vi "Write Variant Cluster to Config File.vi"(5 "Index":i32, 7 "From Array?":bool, 8 "error in":errorcluster, 10 "Variant Configuration Object":variant, 11 "Config Refnum in":T1) -> (0 "error out":errorcluster, 3 "Config Refnum out":T1)   [LabVIEW 2018, in "EMS Generic Actor.lvlib" / "EMS Generic.lvclass"]
doc: "This VI accepts either a Cluster or Array of Clusters that has been converted to a variant. The label of the cluster is used to define the section name and individual control names are used to define key names."
uses:
  EMS Generic.lvclass
  <vilib>/Utility/config.llb/Config Data RefNum.ctl
  <vilib>/Utility/config.llb/Write Key (String).vi
  <vilib>/Utility/config.llb/Write Key (Double).vi
  <vilib>/Utility/config.llb/Write Key (U32).vi
  <vilib>/Utility/config.llb/Write Key (I32).vi
  <vilib>/Utility/config.llb/Write Key (Path).vi
  <vilib>/Utility/Data Type/NI_Data Type.lvlib
  <vilib>/Utility/config.llb/NI_LVConfig.lvlib
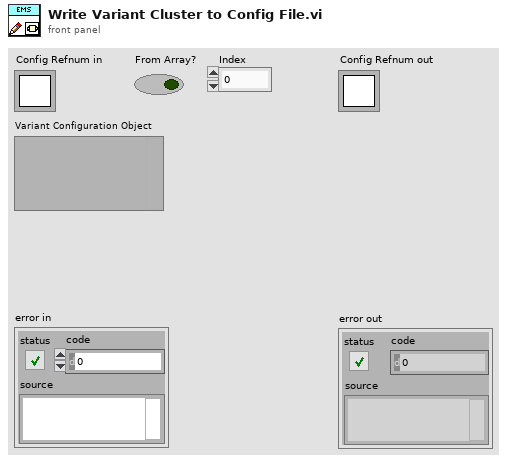
[diagram p1: front panel]
types:
  T1 = typedef "NI_LVConfig.lvlib/Config Data RefNum.ctl" = refnum<k1>
  T2 = typedef "NI_Data Type.lvlib/Data Type.ctl" = enum8{"Invalid Type", "Void", "I8", "I16", "I32", "I64", "U8", "U16", "U32", "U64", "Single Float", "Double Float", "Extended Float", "Single Complex", "Double Complex", "Extended Complex", "Enum U8", "Enum U16", "Enum U32", "Enum U64", "Single Float With Unit", "Double Float With Unit", "Extended Float With Unit", "Single Complex with Unit", "Double Complex with Unit", "Extended Complex with Unit", "Boolean", "String", "Path", "Picture", "Tag", "Array", "Cluster", "Variant", "LV Variant", "Waveform", "Timestamp", "Digital Waveform", "Digital Data", "ExpressData", "Refnum", "External Data", "VI", "Poly VI", "LabVIEW Class Instance", "Fixed Point"}
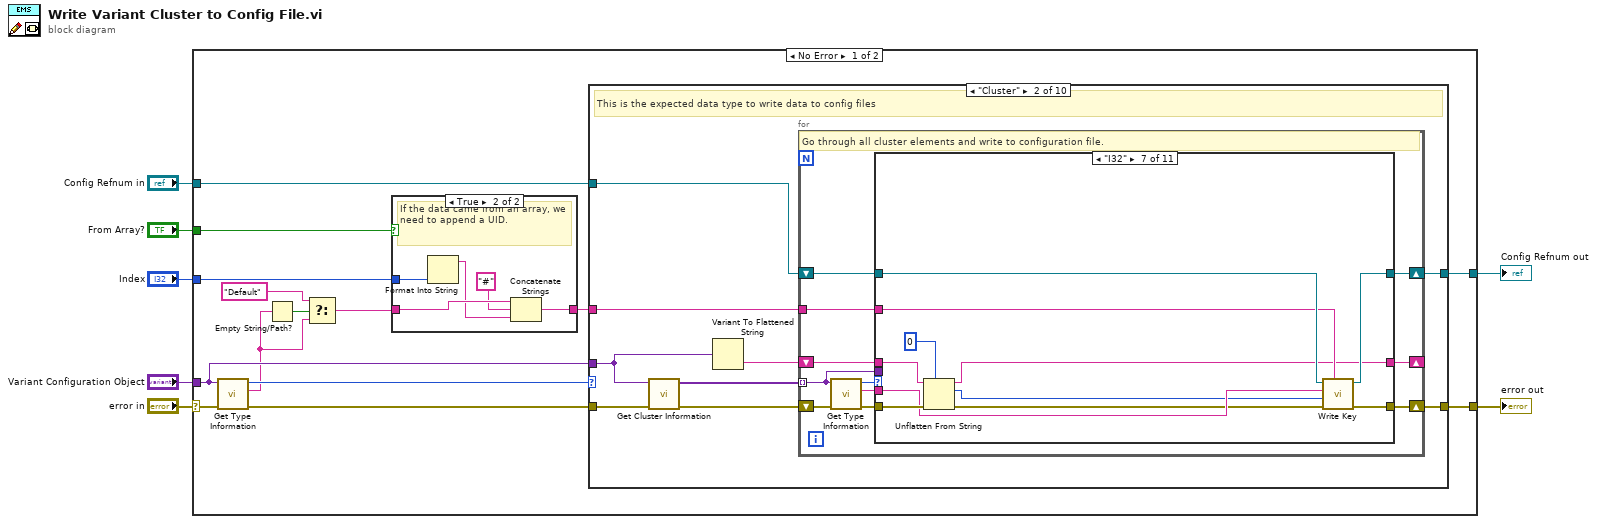
[diagram p0: block diagram]
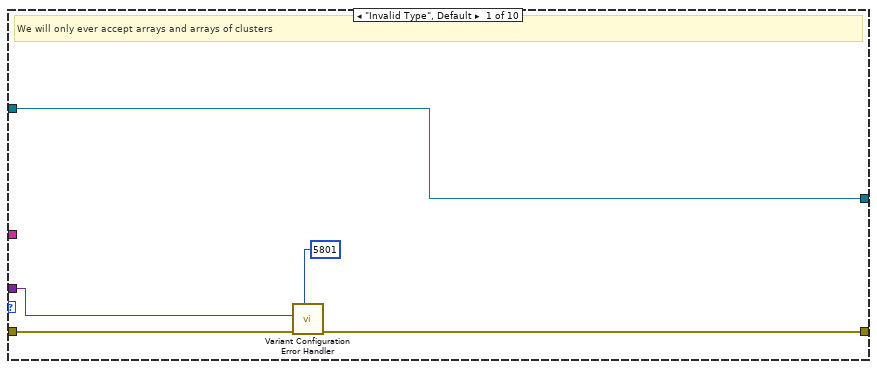
[diagram p2: hidden frame]
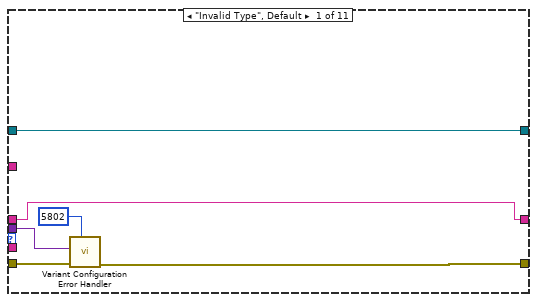
[diagram p3: hidden frame]
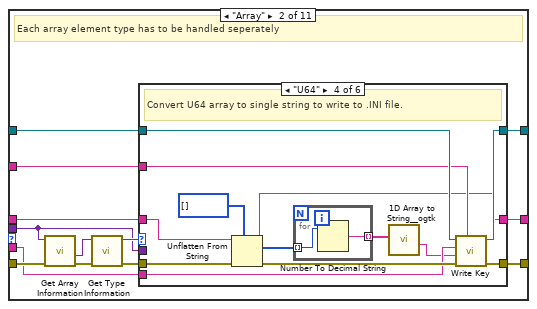
[diagram p4: hidden frame]
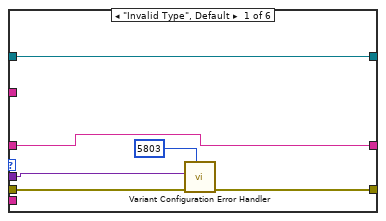
[diagram p5: hidden frame]
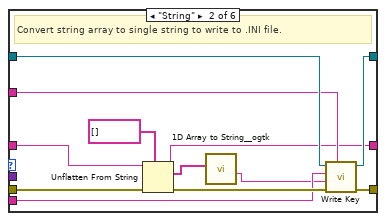
[diagram p6: hidden frame]
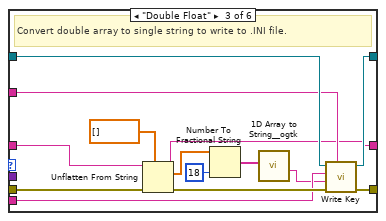
[diagram p7: hidden frame]
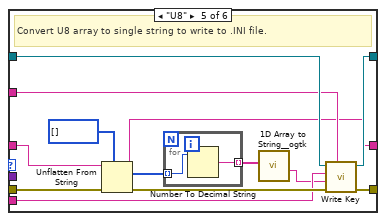
[diagram p8: hidden frame]
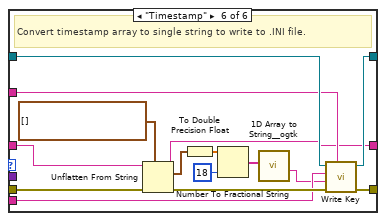
[diagram p9: hidden frame]
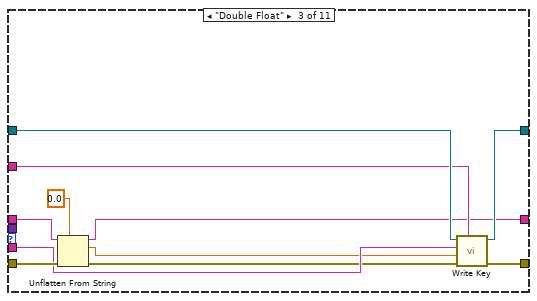
[diagram p10: hidden frame]
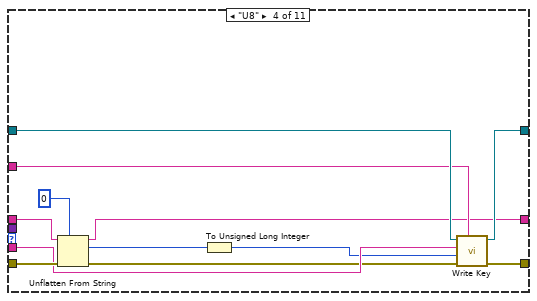
[diagram p11: hidden frame]
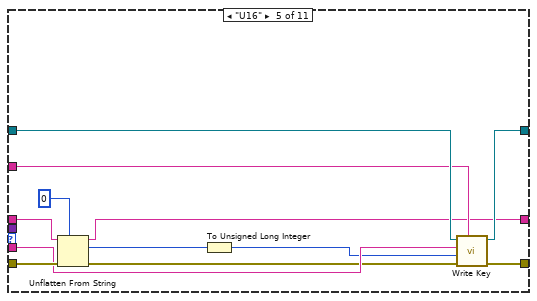
[diagram p12: hidden frame]
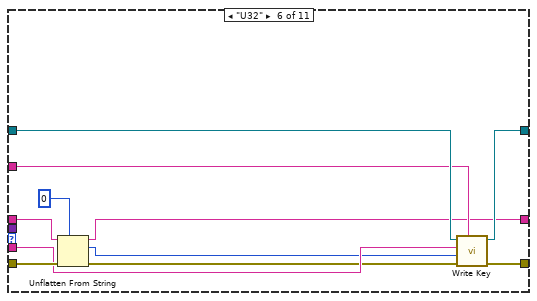
[diagram p13: hidden frame]
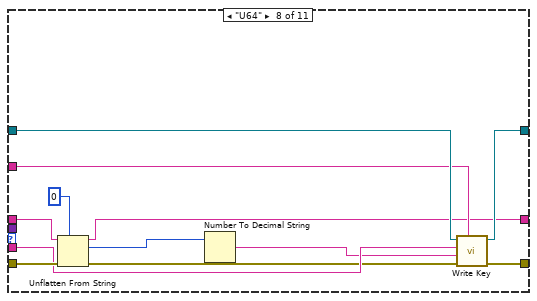
[diagram p14: hidden frame]
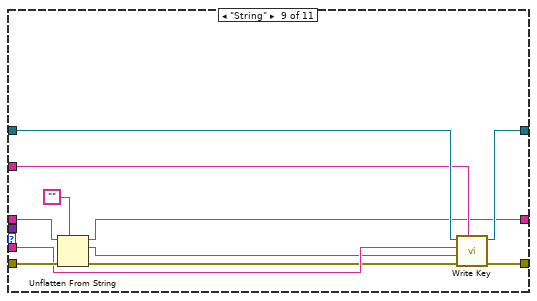
[diagram p15: hidden frame]
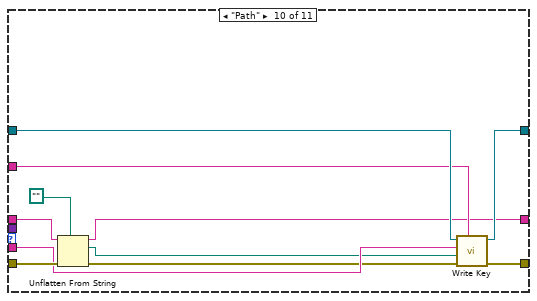
[diagram p16: hidden frame]
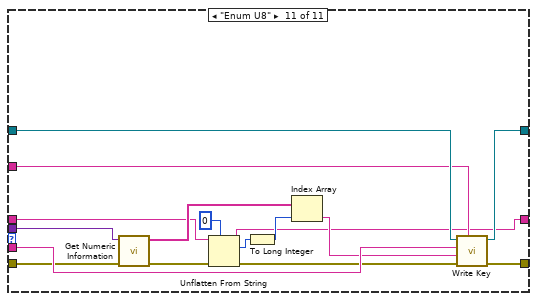
[diagram p17: hidden frame]
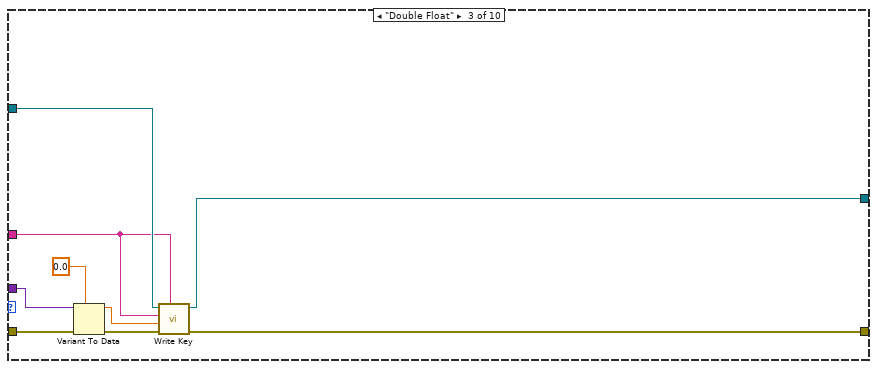
[diagram p18: hidden frame]
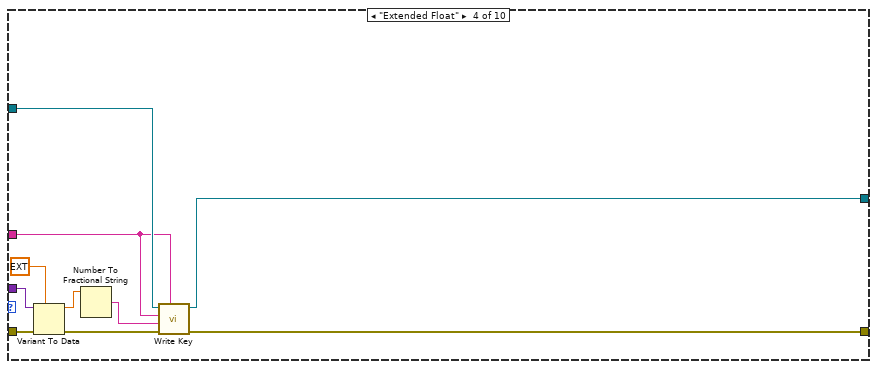
[diagram p19: hidden frame]
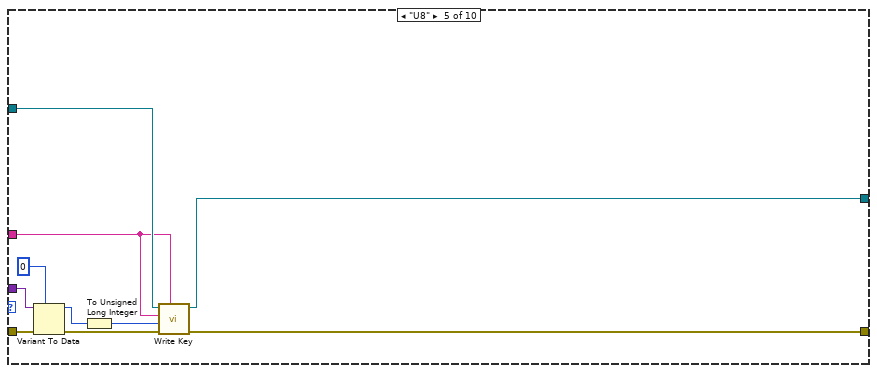
[diagram p20: hidden frame]
diagram:
  n1 = case shown="No Error" "error in" {
    selector: "error in" -> [w21 w340]
    tunnel: "Variant Configuration Object" -> [w19 _]
    tunnel: "Config Refnum in" -> [w17 w341]
    tunnel: "Index" -> [w13 _]
    tunnel: "From Array?" -> [w12 _]
    tunnel: [w16 w341] -> w2
    tunnel: [w15 w340] -> w1
    frame No Error {
      n2 = call <vilib>:"Get Type Information.vi"("error in (no error)"=w21, "Variant"=w19) -> ("error out"=w18:errorcluster, "Name"=w10:string, "Type"=w20:T2)  [unwired: 5 in, 2 out]
      n3 = Empty String/Path?(string/path=w10) -> (empty?=w11:bool)
      n4 = Select(t="Default", s=w11, f=w10) -> (s? t:f=w9:string)
      n5 = case shown="True" w12 {
        tunnel: w9 -> [w334 w338]
        tunnel: [w334 w335] -> w14
        tunnel: w13 -> [_ w339]
        frame False {
          # "Pass the name through as the section name."
        }
        frame True {
          # "If the data came from an array, we need to append a UID."
          n6 = Format Into String(w339) -> (resulting string=w336:string)  [unwired: 3 in, 1 out]
          n7 = Concatenate Strings(w338, "#" ("string"), w336) -> (w335:string)
        }
      }
      n8 = case shown="\"Cluster\"" w20 {
        tunnel: w19 -> [w24 w29 w255 w265 w275 w285 w294 w304 w313 w325]
        tunnel: w18 -> [w26 w35 w253 w263 w273 w283 w292 w302 w311 w326]
        tunnel: [w25 w33 w256 w266 w276 w286 w295 w305 w314 w320] -> w15
        tunnel: w17 -> [w22 w31 w258 w268 w278 w288 w297 w307 w316 w319]
        tunnel: [w22 w30 w257 w267 w277 w287 w296 w306 w315 w317] -> w16
        tunnel: w14 -> [_ w27 w250 w259 w269 w279 w289 w298 w308 _]
        frame "Invalid Type", Default {
          # "We will only ever accept arrays and arrays of clusters"
          n9 = call "Variant Configuration Error Handler.vi"("Error Code"=5801 ("error code (0)"), "error in"=w26, "Variant"=w24) -> ("error out"=w25:errorcluster)  [unwired: 8 in]
        }
        frame "Cluster" {
          # "This is the expected data type to write data to config files"
          n10 = call <vilib>:"Get Cluster Information.vi"("error in (no error)"=w35, "Variant"=w29) -> ("error out"=w34:errorcluster, "Cluster Elements"=w32:variant[])  [unwired: 8 in]
          n11 = Variant To Flattened String(Variant=w29) -> (data string=w28:string)  [unwired: 1 out]
          n12 = for {
            shift-right: [w43] -> w33
            shift-left: w34 -> [w46]
            tunnel: w32 -> [w36] mode=indexing
            tunnel: w27 -> [w41]
            shift-right: [w39] -> w30
            shift-left: w31 -> [w42]
            shift-right: [w37] -> _
            shift-left: w28 -> [w38]
            # "Go through all cluster elements and write to configuration file."
            n13 = call <vilib>:"Get Type Information.vi"("error in (no error)"=w46, "Variant"=w36) -> ("error out"=w44:errorcluster, "Name"=w40:string, "Type"=w45:T2)  [unwired: 5 in, 2 out]
            n14 = case shown="\"I32\"" w45 {
              tunnel: w44 -> [w51 w65 w153 w165 w177 w188 w199 w211 w222 w233 w242]
              tunnel: [w50 w58 w147 w159 w171 w182 w193 w204 w217 w228 w244] -> w43
              tunnel: w42 -> [w49 w60 w151 w163 w175 w186 w197 w209 w221 w232 w248]
              tunnel: w41 -> [_ w59 w150 w162 w174 w185 w196 w208 w220 w231 w247]
              tunnel: w40 -> [_ w57 w149 w161 w173 w184 w195 w207 w219 w230 w246]
              tunnel: [w49 w56 w146 w157 w169 w181 w192 w203 w216 w227 w243] -> w39
              tunnel: w38 -> [w48 w55 w144 w154 w166 w178 w189 w202 w215 w226 w235]
              tunnel: [w48 w54 w143 w155 w167 w179 w190 w201 w214 w225 w234] -> w37
              tunnel: w36 -> [w47 w53 _ _ _ _ _ _ _ _ w237]
              frame "Invalid Type", Default {
                n15 = call "Variant Configuration Error Handler.vi"("Error Code"=5802 ("error code (0)"), "error in"=w51, "Variant"=w47) -> ("error out"=w50:errorcluster)  [unwired: 8 in]
              }
              frame "Array" {
                # "Each array element type has to be handled seperately"
                n16 = call <vilib>:"Get Array Information.vi"("error in (no error)"=w65, "Variant"=w53) -> ("error out"=w63:errorcluster, "Array Element Data Type"=w62:variant)  [unwired: 6 in, 2 out]
                n17 = call <vilib>:"Get Type Information.vi"("error in (no error)"=w63, "Variant"=w62) -> ("error out"=w61:errorcluster, "Type"=w64:T2)  [unwired: 5 in, 3 out]
                n18 = case shown="\"U64\"" w64 {
                  tunnel: w61 -> [w70 w83 w97 w110 w125 w142]
                  tunnel: w60 -> [w68 w79 w93 w106 w121 w138]
                  tunnel: w59 -> [_ w78 w92 w105 w120 w137]
                  tunnel: [w69 w80 w94 w107 w122 w139] -> w58
                  tunnel: w57 -> [_ w77 w91 w104 w119 w136]
                  tunnel: [w68 w75 w87 w102 w117 w131] -> w56
                  tunnel: w55 -> [w67 w73 w85 w101 w116 w130]
                  tunnel: [w67 w72 w84 w100 w115 w128] -> w54
                  tunnel: w53 -> [w66 _ _ _ _ _]
                  frame "Invalid Type", Default {
                    n19 = call "Variant Configuration Error Handler.vi"("Error Code"=5803 ("error code (0)"), "error in"=w70, "Variant"=w66) -> ("error out"=w69:errorcluster)  [unwired: 8 in]
                  }
                  frame "String" {
                    # "Convert string array to single string to write to .INI file."
                    n20 = Unflatten From String(type=string[] [], binary string=w73, error in (no error)=w83) -> (rest of the binary string=w72:string, value=w74:string[], error out=w81:errorcluster)  [unwired: 2 in]
                    n21 = call <userlib>:"1D Array to String__ogtk.vi"("Array of Strings"=w74) -> ("delimited string"=w76:string)  [unwired: 10 in]
                    n22 = call-poly <vilib>:"Write Key.vi"("section"=w78, "error in (no error)"=w81, "value"=w76, "key"=w77, "refnum"=w79) -> ("error out"=w80:errorcluster, "refnum out"=w75:T1)  [unwired: 4 in, 1 out]
                  }
                  frame "Double Float" {
                    # "Convert double array to single string to write to .INI file."
                    n23 = Unflatten From String(type=dbl[] [], binary string=w85, error in (no error)=w97) -> (rest of the binary string=w84:string, value=w86:dbl[], error out=w95:errorcluster)  [unwired: 2 in]
                    n24 = Number To Fractional String(number=w86, precision (6)=i16 18) -> (F-format string=w89:string[])  [unwired: 2 in]
                    n25 = call <userlib>:"1D Array to String__ogtk.vi"("Array of Strings"=w89) -> ("delimited string"=w88:string)  [unwired: 10 in]
                    n26 = call-poly <vilib>:"Write Key.vi"("section"=w92, "error in (no error)"=w95, "value"=w88, "key"=w91, "refnum"=w93) -> ("error out"=w94:errorcluster, "refnum out"=w87:T1)  [unwired: 4 in, 1 out]
                  }
                  frame "U64" {
                    # "Convert U64 array to single string to write to .INI file."
                    n27 = Unflatten From String(type=u64[] [], binary string=w101, error in (no error)=w110) -> (rest of the binary string=w100:string, value=w99:u64[], error out=w108:errorcluster)  [unwired: 2 in]
                    n28 = for {
                      tunnel: w99 -> [w112] mode=indexing
                      tunnel: [w111] -> w98 mode=indexing
                      n29 = Number To Decimal String(number=w112) -> (decimal integer string=w111:string)  [unwired: 1 in]
                    }
                    n30 = call <userlib>:"1D Array to String__ogtk.vi"("Array of Strings"=w98) -> ("delimited string"=w103:string)  [unwired: 10 in]
                    n31 = call-poly <vilib>:"Write Key.vi"("section"=w105, "error in (no error)"=w108, "value"=w103, "key"=w104, "refnum"=w106) -> ("error out"=w107:errorcluster, "refnum out"=w102:T1)  [unwired: 4 in, 1 out]
                  }
                  frame "U8" {
                    # "Convert U8 array to single string to write to .INI file."
                    n32 = Unflatten From String(type=u8[] [], binary string=w116, error in (no error)=w125) -> (rest of the binary string=w115:string, value=w114:u8[], error out=w123:errorcluster)  [unwired: 2 in]
                    n33 = for {
                      tunnel: w114 -> [w127] mode=indexing
                      tunnel: [w126] -> w113 mode=indexing
                      n34 = Number To Decimal String(number=w127) -> (decimal integer string=w126:string)  [unwired: 1 in]
                    }
                    n35 = call <userlib>:"1D Array to String__ogtk.vi"("Array of Strings"=w113) -> ("delimited string"=w118:string)  [unwired: 10 in]
                    n36 = call-poly <vilib>:"Write Key.vi"("section"=w120, "error in (no error)"=w123, "value"=w118, "key"=w119, "refnum"=w121) -> ("error out"=w122:errorcluster, "refnum out"=w117:T1)  [unwired: 4 in, 1 out]
                  }
                  frame "Timestamp" {
                    # "Convert timestamp array to single string to write to .INI file."
                    n37 = Unflatten From String(type=timestamp[] [], binary string=w130, error in (no error)=w142) -> (rest of the binary string=w128:string, value=w129:timestamp[], error out=w140:errorcluster)  [unwired: 2 in]
                    n38 = To Double Precision Float(number=w129) -> (double precision float=w132:dbl[])
                    n39 = Number To Fractional String(number=w132, precision (6)=i16 18) -> (F-format string=w134:string[])  [unwired: 2 in]
                    n40 = call <userlib>:"1D Array to String__ogtk.vi"("Array of Strings"=w134) -> ("delimited string"=w133:string)  [unwired: 10 in]
                    n41 = call-poly <vilib>:"Write Key.vi"("section"=w137, "error in (no error)"=w140, "value"=w133, "key"=w136, "refnum"=w138) -> ("error out"=w139:errorcluster, "refnum out"=w131:T1)  [unwired: 4 in, 1 out]
                  }
                }
              }
              frame "Double Float" {
                n42 = Unflatten From String(type=0.0, binary string=w144, error in (no error)=w153) -> (rest of the binary string=w143:string, value=w145:dbl, error out=w148:errorcluster)  [unwired: 2 in]
                n43 = call-poly <vilib>:"Write Key.vi"("section"=w150, "error in (no error)"=w148, "value"=w145, "key"=w149, "refnum"=w151) -> ("error out"=w147:errorcluster, "refnum out"=w146:T1)  [unwired: 4 in, 1 out]
              }
              frame "U8" {
                n44 = Unflatten From String(type=u8 0, binary string=w154, error in (no error)=w165) -> (rest of the binary string=w155:string, value=w156:u8, error out=w160:errorcluster)  [unwired: 2 in]
                n45 = To Unsigned Long Integer(number=w156) -> (unsigned 32bit integer=w158:u32)
                n46 = call-poly <vilib>:"Write Key.vi"("section"=w162, "error in (no error)"=w160, "value"=w158, "key"=w161, "refnum"=w163) -> ("error out"=w159:errorcluster, "refnum out"=w157:T1)  [unwired: 4 in, 1 out]
              }
              frame "U16" {
                n47 = Unflatten From String(type=u16 0, binary string=w166, error in (no error)=w177) -> (rest of the binary string=w167:string, value=w168:u16, error out=w172:errorcluster)  [unwired: 2 in]
                n48 = To Unsigned Long Integer(number=w168) -> (unsigned 32bit integer=w170:u32)
                n49 = call-poly <vilib>:"Write Key.vi"("section"=w174, "error in (no error)"=w172, "value"=w170, "key"=w173, "refnum"=w175) -> ("error out"=w171:errorcluster, "refnum out"=w169:T1)  [unwired: 4 in, 1 out]
              }
              frame "U32" {
                n50 = Unflatten From String(type=u32 0, binary string=w178, error in (no error)=w188) -> (rest of the binary string=w179:string, value=w180:u32, error out=w183:errorcluster)  [unwired: 2 in]
                n51 = call-poly <vilib>:"Write Key.vi"("section"=w185, "error in (no error)"=w183, "value"=w180, "key"=w184, "refnum"=w186) -> ("error out"=w182:errorcluster, "refnum out"=w181:T1)  [unwired: 4 in, 1 out]
              }
              frame "I32" {
                n52 = Unflatten From String(type=0, binary string=w189, error in (no error)=w199) -> (rest of the binary string=w190:string, value=w191:i32, error out=w194:errorcluster)  [unwired: 2 in]
                n53 = call-poly <vilib>:"Write Key.vi"("section"=w196, "error in (no error)"=w194, "value"=w191, "key"=w195, "refnum"=w197) -> ("error out"=w193:errorcluster, "refnum out"=w192:T1)  [unwired: 4 in, 1 out]
              }
              frame "U64" {
                n54 = Unflatten From String(type=u64 0, binary string=w202, error in (no error)=w211) -> (rest of the binary string=w201:string, value=w200:u64, error out=w205:errorcluster)  [unwired: 2 in]
                n55 = Number To Decimal String(number=w200) -> (decimal integer string=w206:string)  [unwired: 1 in]
                n56 = call-poly <vilib>:"Write Key.vi"("section"=w208, "error in (no error)"=w205, "value"=w206, "key"=w207, "refnum"=w209) -> ("error out"=w204:errorcluster, "refnum out"=w203:T1)  [unwired: 4 in, 1 out]
              }
              frame "String" {
                n57 = Unflatten From String(type="", binary string=w215, error in (no error)=w222) -> (rest of the binary string=w214:string, value=w213:string, error out=w218:errorcluster)  [unwired: 2 in]
                n58 = call-poly <vilib>:"Write Key.vi"("section"=w220, "error in (no error)"=w218, "value"=w213, "key"=w219, "refnum"=w221) -> ("error out"=w217:errorcluster, "refnum out"=w216:T1)  [unwired: 4 in, 1 out]
              }
              frame "Path" {
                n59 = Unflatten From String(type=path "", binary string=w226, error in (no error)=w233) -> (rest of the binary string=w225:string, value=w224:path, error out=w229:errorcluster)  [unwired: 2 in]
                n60 = call-poly <vilib>:"Write Key.vi"("section"=w231, "error in (no error)"=w229, "value"=w224, "key"=w230, "refnum"=w232) -> ("error out"=w228:errorcluster, "refnum out"=w227:T1)  [unwired: 4 in, 1 out]
              }
              frame "Enum U8" {
                n61 = call <vilib>:"Get Numeric Information.vi"("error in (no error)"=w242, "Variant"=w237) -> ("error out"=w241:errorcluster, "Enum Names"=w240:string[])  [unwired: 6 in, 2 out]
                n62 = Unflatten From String(type=u8 0, binary string=w235, error in (no error)=w241) -> (rest of the binary string=w234:string, value=w236:u8, error out=w245:errorcluster)  [unwired: 2 in]
                n63 = To Long Integer(number=w236) -> (32bit integer=w239:i32)
                n64 = Index Array(array=w240, index=w239) -> (element=w238:string)
                n65 = call-poly <vilib>:"Write Key.vi"("section"=w247, "error in (no error)"=w245, "value"=w238, "key"=w246, "refnum"=w248) -> ("error out"=w244:errorcluster, "refnum out"=w243:T1)  [unwired: 4 in, 1 out]
              }
            }
          }
        }
        frame "Double Float" {
          n66 = Variant To Data(error in=w253, type=0.0, Variant=w255) -> (data=w251:dbl, error out=w252:errorcluster)
          n67 = call-poly <vilib>:"Write Key.vi"("section"=w250, "error in (no error)"=w252, "value"=w251, "key"=w250, "refnum"=w258) -> ("error out"=w256:errorcluster, "refnum out"=w257:T1)  [unwired: 4 in, 1 out]
        }
        frame "Extended Float" {
          n68 = Variant To Data(error in=w263, type=ext 0.0, Variant=w265) -> (data=w261:ext, error out=w262:errorcluster)
          n69 = Number To Fractional String(number=w261) -> (F-format string=w260:string)  [unwired: 3 in]
          n70 = call-poly <vilib>:"Write Key.vi"("section"=w259, "error in (no error)"=w262, "value"=w260, "key"=w259, "refnum"=w268) -> ("error out"=w266:errorcluster, "refnum out"=w267:T1)  [unwired: 4 in, 1 out]
        }
        frame "U8" {
          n71 = Variant To Data(error in=w273, type=u8 0, Variant=w275) -> (data=w271:u8, error out=w272:errorcluster)
          n72 = To Unsigned Long Integer(number=w271) -> (unsigned 32bit integer=w270:u32)
          n73 = call-poly <vilib>:"Write Key.vi"("section"=w269, "error in (no error)"=w272, "value"=w270, "key"=w269, "refnum"=w278) -> ("error out"=w276:errorcluster, "refnum out"=w277:T1)  [unwired: 4 in, 1 out]
        }
        frame "U16" {
          n74 = Variant To Data(error in=w283, type=u16 0, Variant=w285) -> (data=w281:u16, error out=w282:errorcluster)
          n75 = To Unsigned Long Integer(number=w281) -> (unsigned 32bit integer=w280:u32)
          n76 = call-poly <vilib>:"Write Key.vi"("section"=w279, "error in (no error)"=w282, "value"=w280, "key"=w279, "refnum"=w288) -> ("error out"=w286:errorcluster, "refnum out"=w287:T1)  [unwired: 4 in, 1 out]
        }
        frame "U32" {
          n77 = Variant To Data(error in=w292, type=u32 0, Variant=w294) -> (data=w290:u32, error out=w291:errorcluster)
          n78 = call-poly <vilib>:"Write Key.vi"("section"=w289, "error in (no error)"=w291, "value"=w290, "key"=w289, "refnum"=w297) -> ("error out"=w295:errorcluster, "refnum out"=w296:T1)  [unwired: 4 in, 1 out]
        }
        frame "U64" {
          n79 = Variant To Data(error in=w302, type=u64 0, Variant=w304) -> (data=w300:u64, error out=w301:errorcluster)
          n80 = Number To Decimal String(number=w300) -> (decimal integer string=w299:string)  [unwired: 1 in]
          n81 = call-poly <vilib>:"Write Key.vi"("section"=w298, "error in (no error)"=w301, "value"=w299, "key"=w298, "refnum"=w307) -> ("error out"=w305:errorcluster, "refnum out"=w306:T1)  [unwired: 4 in, 1 out]
        }
        frame "String" {
          n82 = Variant To Data(error in=w311, type="", Variant=w313) -> (data=w309:string, error out=w310:errorcluster)
          n83 = call-poly <vilib>:"Write Key.vi"("section"=w308, "error in (no error)"=w310, "value"=w309, "key"=w308, "refnum"=w316) -> ("error out"=w314:errorcluster, "refnum out"=w315:T1)  [unwired: 4 in, 1 out]
        }
        frame "Array" {
          # "Converts single variant of array of clusters to array of variant clusters."
          # "If its an array we call back into the code to handle each cluster individually."
          n84 = call <vilib>:"Get Array Information.vi"("error in (no error)"=w326, "Variant"=w325) -> ("error out"=w322:errorcluster, "Array Element Data Type"=w324:variant)  [unwired: 6 in, 2 out]
          n85 = Build Array(w324) -> (w323:variant[])
          n86 = Variant To Data(error in=w322, type=w323, Variant=w325) -> (data=w318:variant[], error out=w321:errorcluster)
          n87 = for {
            shift-right: [w332] -> w320
            shift-left: w321 -> [w333]
            tunnel: w318 -> [w330] mode=indexing
            shift-right: [w327] -> w317
            shift-left: w319 -> [w331]
            i -> [w328]
            # "Recursion is awful"
            n88 = call "Write Variant Cluster to Config File.vi"("Index"=w328, "From Array?"=TRUE, "error in"=w333, "Variant Configuration Object"=w330, "Config Refnum in"=w331) -> ("error out"=w332:errorcluster, "Config Refnum out"=w327:T1)  [unwired: 5 in]
          }
        }
      }
    }
    frame Error {
    }
  }
  "error out" <- w1
  "Config Refnum out" <- w2
